vi "Open file.vi"(8 "error in (no error)":errorcluster, 9 "access (0:read/write)":T1, 10 "File Path":path, 11 "AMS Connection":T2) -> (0 "error out":errorcluster, 2 "File Handle":i32, 3 "AMS Connection Out":T2)   [LabVIEW 2017, in "TwinCAT ADS.lvlib" / "System Service.lvlib"]
uses:
  System Service.lvlib
  Low Level/TypeDefs/AMS Connection.ctl
  Low Level/TypeDefs/AMS.ctl
  TypeDefs/Access Mode.ctl
  <vilib>/Utility/error.llb/Error Cluster From Error Code.vi
  <vilib>/ErrorRing/Error Ring.xnode
  TwinCAT ADS.lvlib
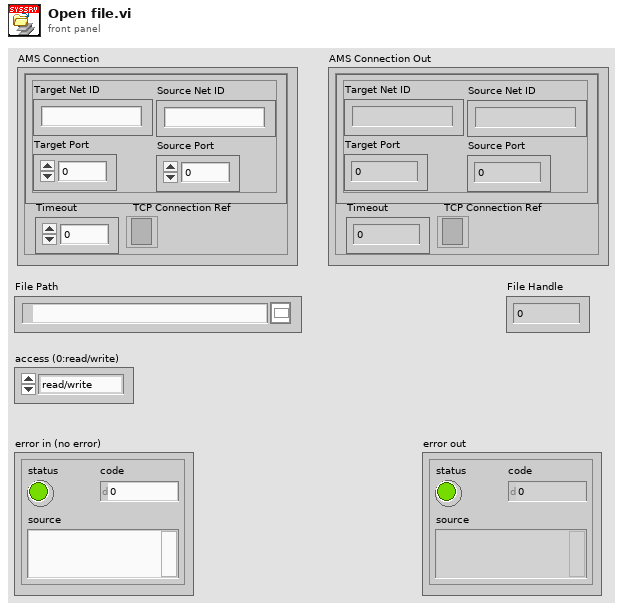
[diagram p1: front panel]
types:
  T1 = typedef "TwinCAT ADS.lvlib/System Service.lvlib/Access Mode.ctl" = enum16{"read/write", "read-only", "write-only"}
  T2 = typedef "TwinCAT ADS.lvlib/AMS Connection.ctl" = cluster{"AMS":T3, "Timeout":i32, "TCP Connection Ref":refnum<k5>}
  T3 = typedef "TwinCAT ADS.lvlib/AMS.ctl" = cluster{"Target Net ID":string, "Target Port":u16, "Source Net ID":string, "Source Port":u16}
  T4 = typedef "TwinCAT ADS.lvlib/ADS Error.ctl" = i32
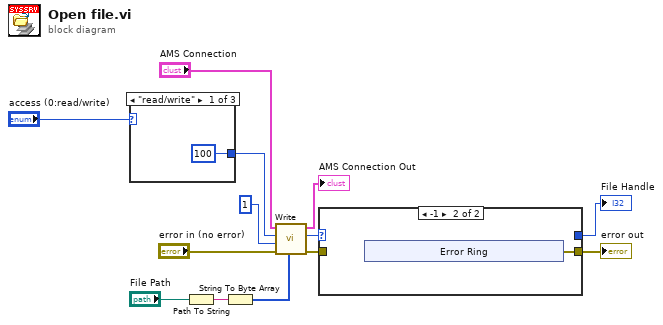
[diagram p0: block diagram]
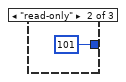
[diagram p3: hidden frame]
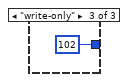
[diagram p4: hidden frame]
diagram:
  n1 = case shown="\"read/write\"" "access (0:read/write)" {
    tunnel: [u32 100 ("Index Group") u32 101 ("Index Group") u32 102 ("Index Group")] -> w5
    frame "read/write" {
    }
    frame "read-only" {
    }
    frame "write-only" {
    }
  }
  n2 = Path To String(path="File Path") -> (string=w7:string)
  n3 = String To Byte Array(string=w7) -> (unsigned byte array=w12:u8[])
  n4 = call "Write.vi"("Data"=w12, "Error In"="error in (no error)", "Offset"=u32 1, "Index Group"=w5, "AMS Connection In"="AMS Connection") -> ("Error Out"=w3:errorcluster, "ADS Error"=w2:T4, "AMS Connection Out"=→"AMS Connection Out":T2)  [unwired: 4 in]
  n5 = case shown="-1" w2 {
    selector: w2 -> [w17 _]
    tunnel: [w18 w19] -> w4
    tunnel: w3 -> [w18 _]
    tunnel: [w17 _] -> w1
    frame Default {
    }
    frame -1 {
      n6 = xnode "Error Ring"() -> ("error out"=w19:errorcluster)
    }
  }
  "error out" <- w4
  "File Handle" <- w1
